vi "PushOpenSet.vi"(9 "Novo nó":dbl[](array[numeric]), 10 "OpenSet":dbl[][](array[numeric])) -> (2 "NewOpenSet":dbl[][](array[numeric]))   [LabVIEW 2016]
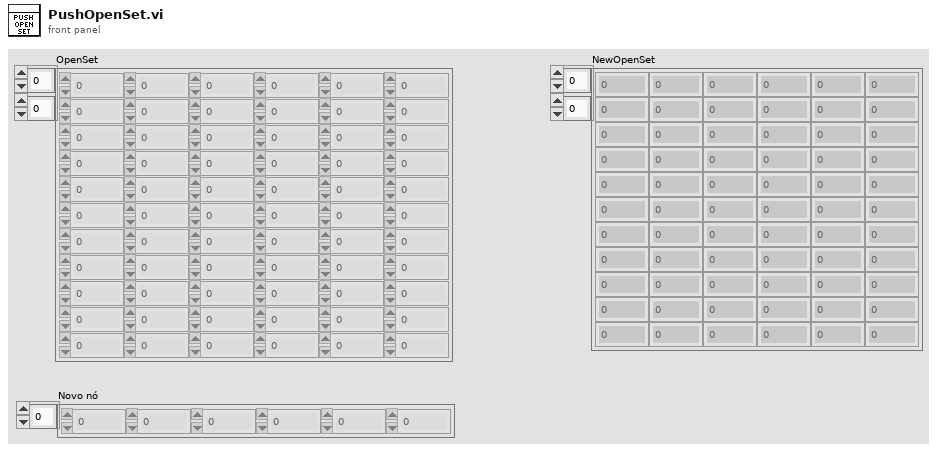
[diagram p1: front panel]
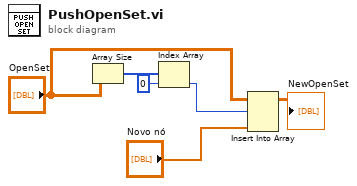
[diagram p0: block diagram]
diagram:
  n1 = Array Size(array="OpenSet") -> (size(s)=w6:i32[])
  n2 = Index Array(array=w6, index=0) -> (element=w4:i32)
  n3 = Insert Into Array(array="OpenSet", index (row)=w4, new element="Novo nó") -> (→"NewOpenSet":dbl[][])  [unwired: 1 in]
